vi "Read Min Max Vectors.vi"(0 "TDMS In":refnum<k34>, 11 "Error In":errorcluster) -> (2 "Inputs Min":dbl[](array[numeric]), 3 "Inputs Max":dbl[](array[numeric]), 4 "TDMS Out":refnum<k34>, 13 "Outputs Min":dbl[](array[numeric]), 14 "Outputs Max":dbl[](array[numeric]), 15 "Error Out":errorcluster)   [LabVIEW 2015, in "Teaching File.lvlib"]
doc: "Read the min and max vectors for each IO channel."
uses:
  Teaching File.lvlib
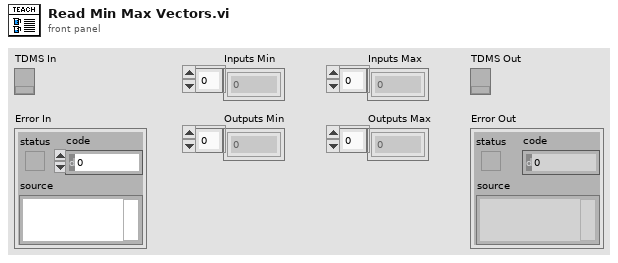
[diagram p1: front panel]
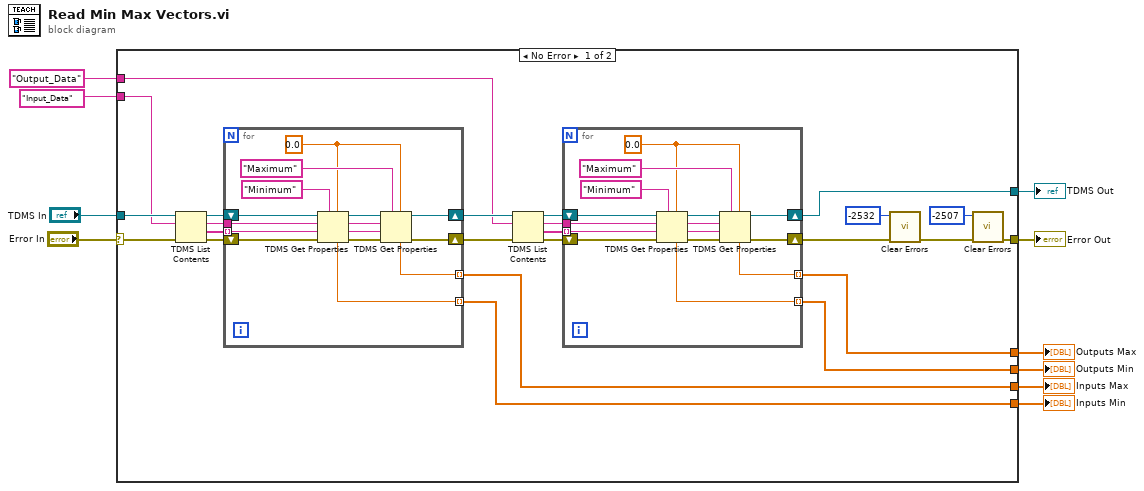
[diagram p0: block diagram]
diagram:
  n1 = case shown="No Error" "Error In" {
    selector: "Error In" -> [w29 w66]
    tunnel: "TDMS In" -> [w34 w65]
    tunnel: [w30 w66] -> w9
    tunnel: [w19 w65] -> w7
    tunnel: [w13 _] -> w6
    tunnel: [w14 _] -> w5
    tunnel: [w11 _] -> w4
    tunnel: [w12 _] -> w3
    tunnel: "Input_Data" ("group name") -> [w17 _]
    tunnel: "Output_Data" ("group name") -> [w16 _]
    frame No Error {
      n2 = TDMS List Contents(4:w29, 6:w17, 7:w34) -> (0:w27:errorcluster, 1:w25:string[], 2:w26:string, 3:w28:refnum<k34>)
      n3 = for {
        tunnel: w26 -> [w47]
        tunnel: w25 -> [w46] mode=indexing
        tunnel: [w44] -> w12 mode=indexing
        shift-right: [w36] -> w24
        shift-left: w28 -> [w49]
        shift-right: [w35] -> w18
        shift-left: w27 -> [w48]
        tunnel: [w37] -> w11 mode=indexing
        w38 = 0.0
        n4 = TDMS Get Properties(5:w38, 7:"Minimum" ("group name in"), 8:w48, 9:w46, 10:w47, 11:w49) -> (0:w40:errorcluster, 1:w41:string, 2:w42:string, 3:w43:refnum<k34>, 4:w44:dbl)  [unwired: 1 out]
        n5 = TDMS Get Properties(5:w38, 7:"Maximum" ("group name in"), 8:w40, 9:w41, 10:w42, 11:w43) -> (0:w35:errorcluster, 3:w36:refnum<k34>, 4:w37:dbl)  [unwired: 3 out]
      }
      n6 = TDMS List Contents(4:w18, 6:w16, 7:w24) -> (0:w20:errorcluster, 1:w21:string[], 2:w22:string, 3:w23:refnum<k34>)
      n7 = for {
        tunnel: w22 -> [w62]
        tunnel: w21 -> [w61] mode=indexing
        tunnel: [w59] -> w14 mode=indexing
        shift-right: [w51] -> w19
        shift-left: w23 -> [w64]
        shift-right: [w50] -> w15
        shift-left: w20 -> [w63]
        tunnel: [w52] -> w13 mode=indexing
        w53 = 0.0
        n8 = TDMS Get Properties(5:w53, 7:"Minimum" ("group name in"), 8:w63, 9:w61, 10:w62, 11:w64) -> (0:w55:errorcluster, 1:w56:string, 2:w57:string, 3:w58:refnum<k34>, 4:w59:dbl)  [unwired: 1 out]
        n9 = TDMS Get Properties(5:w53, 7:"Maximum" ("group name in"), 8:w55, 9:w56, 10:w57, 11:w58) -> (0:w50:errorcluster, 3:w51:refnum<k34>, 4:w52:dbl)  [unwired: 3 out]
      }
      n10 = call <vilib>:"Clear Errors.vi"("error in (no error)"=w15, "specific error code to clear (0: all)"=-2532) -> ("error out"=w32:errorcluster)  [unwired: 4 in, 1 out]
      n11 = call <vilib>:"Clear Errors.vi"("error in (no error)"=w32, "specific error code to clear (0: all)"=-2507) -> ("error out"=w30:errorcluster)  [unwired: 4 in, 1 out]
    }
    frame Error {
    }
  }
  "Error Out" <- w9
  "TDMS Out" <- w7
  "Outputs Min" <- w5
  "Outputs Max" <- w6
  "Inputs Min" <- w3
  "Inputs Max" <- w4
